vi "Client Download and Print PDF.vi"(8 "error in (no error)":errorcluster, 11 "PDF URL (\"\")":string) -> (0 "error out":errorcluster)   [LabVIEW 2011]
uses:
  Summitek EXT/Win32/WinSHELL/SHFolderPaths.ctl
  Spartan Client Version.vi
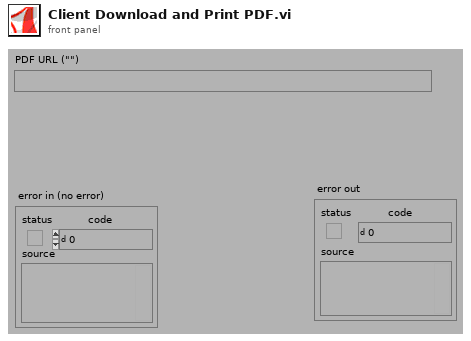
[diagram p1: front panel]
types:
  T1 = typedef "SHFolderPaths.ctl" = i32
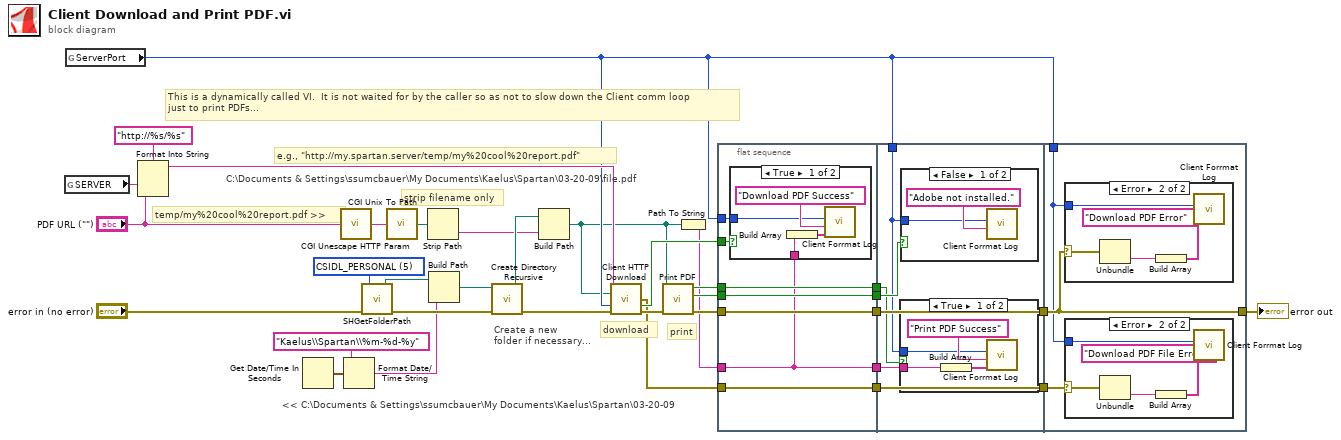
[diagram p0: block diagram]
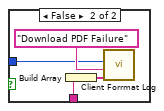
[diagram p2: hidden frame]
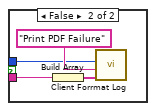
[diagram p3: hidden frame]
diagram:
  w34 = T1 5 items=["CSIDL_DESKTOP"=0, "CSIDL_PERSONAL"=5, "CSIDL_STARTUP"=7, "CSIDL_BITBUCKET"=10, "CSIDL_DRIVES"=17, "CSIDL_NETWORK"=18, "CSIDL_COMMON_PROGRAMS"=23, "CSIDL_COMMON_STARTUP"=24, "CSIDL_COMMON_DESKTOPDIRECTORY"=25, "CSIDL_PROGRAM_FILES"=38] ("Shell Folder (DESKTOP)")
  # "print"
  # "temp/my%20cool%20report.pdf >>"
  # "strip filename only"
  # "e.g., \"http://my.spartan.server/temp/my%20cool%20report.pdf\""
  # "download"
  # "This is a dynamically called VI.  It is not waited for by the caller so as not to slow down the Client comm loop\njust to print PDFs..."
  # "<< C:\\Documents & Settings\\ssumcbauer\\My Documents\\Kaelus\\Spartan\\03-20-09"
  # "C:\\Documents & Settings\\ssumcbauer\\My Documents\\Kaelus\\Spartan\\03-20-09\\file.pdf"
  # "Create a new\nfolder if necessary..."
  n1 = global read "Spartan Client Version.vi" "SERVER"() -> (w7:string)
  n2 = global read "Spartan Client Version.vi" "ServerPort"() -> (w6:u16)
  n3 = Format Into String(format string="http://%s/%s" ("name (unnamed)"), w7, "PDF URL (\"\")") -> (resulting string=w22:string)  [unwired: 2 in, 1 out]
  n4 = Get Date/Time In Seconds() -> (seconds since 1Jan1904=w31:timestamp)
  n5 = call "CGI Unescape HTTP Param.vi"("url-encoded string"="PDF URL (\"\")") -> ("string"=w19:string)
  n6 = Format Date/Time String(time format string (%c)="Kaelus\\Spartan\\%m-%d-%y", seconds (now)=w31) -> (date/time string=w29:string)  [unwired: 1 out]
  n7 = call "SHGetFolderPath.vi"("error in (no error)"="error in (no error)", "Shell Folder (DESKTOP)"=w34) -> ("error out"=w33:errorcluster, "FolderPath"=w32:path)  [unwired: 4 out]
  n8 = call "CGI Unix To Path.vi"("unix path"=w19) -> ("platform path"=w24:path)  [unwired: 1 out]
  n9 = Strip Path(path=w24) -> (name=w21:string)  [unwired: 1 out]
  n10 = Build Path(base path=w32, name or relative path=w29) -> (appended path=w28:path)
  n11 = call <vilib>:"Create Directory Recursive.vi"("error in (no error)"=w33, "directory"=w28) -> ("error out"=w26:errorcluster, "directory copy"=w27:path)  [unwired: 1 in, 3 out]
  n12 = Build Path(base path=w27, name or relative path=w21) -> (appended path=w5:path)
  n13 = call "Client HTTP Download.vi"("http URL"=w22, "file path (Not A Path)"=w5, "Port (80)"=w6, "error in (no error)"=w26) -> ("file error"=w12:errorcluster, "success"=w18:bool, "error out"=w25:errorcluster)  [unwired: 1 in, 8 out]
  n14 = call "Print PDF.vi"("error in (no error)"=w25, "PDF Path"=w5) -> ("error out"=w16:errorcluster, "Adobe Installed?"=w13:bool, "Printed?"=w3:bool)  [unwired: 7 out]
  n15 = Path To String(path=w5) -> (string=w1:string)
  n16 = flat-sequence {
    tunnel: w18 -> [w41]
    tunnel: [w40] -> w17
    tunnel: w16 -> [w40]
    tunnel: [w39] -> w14
    tunnel: w13 -> [w39]
    tunnel: w12 -> [w38]
    tunnel: [w38] -> w11
    tunnel: w6 -> [w37]
    tunnel: [w36] -> w4
    tunnel: w3 -> [w36]
    tunnel: [w35] -> w2
    tunnel: w1 -> [w35]
    tunnel: w17 -> [w55]
    tunnel: [w55] -> w15
    tunnel: w14 -> [w54]
    tunnel: w11 -> [w53]
    tunnel: [w53] -> w10
    tunnel: w6 -> [w51]
    tunnel: w4 -> [w52]
    tunnel: w2 -> [w50]
    tunnel: w15 -> [w68]
    tunnel: [w68] -> w9
    tunnel: w10 -> [w67]
    tunnel: w6 -> [w66]
    frame #0 {
      n17 = case shown="True" w41 {
        tunnel: w37 -> [w43 w48]
        tunnel: w35 -> [w42 w46]
        frame True {
          n18 = Build Array(w42) -> (w44:string[])
          n19 = call "Client Forrmat Log.vi"("Params (empty)"=w44, "Command (\"\")"="Download PDF Success", "ServerPort (80)"=w43) -> ()  [unwired: 1 in, 8 out]
        }
        frame False {
          n20 = Build Array(w46) -> (w47:string[])
          n21 = call "Client Forrmat Log.vi"("Params (empty)"=w47, "Command (\"\")"="Download PDF Failure", "ServerPort (80)"=w48) -> ()  [unwired: 1 in, 8 out]
        }
      }
    }
    frame #1 {
      n22 = case shown="True" w52 {
        tunnel: w51 -> [w57 w61]
        tunnel: w50 -> [w56 w60]
        frame True {
          n23 = Build Array(w56) -> (w58:string[])
          n24 = call "Client Forrmat Log.vi"("Params (empty)"=w58, "Command (\"\")"="Print PDF Success", "ServerPort (80)"=w57) -> ()  [unwired: 1 in, 8 out]
        }
        frame False {
          n25 = Build Array(w60) -> (w62:string[])
          n26 = call "Client Forrmat Log.vi"("Params (empty)"=w62, "Command (\"\")"="Print PDF Failure", "ServerPort (80)"=w61) -> ()  [unwired: 1 in, 8 out]
        }
      }
      n27 = case shown="False" w54 {
        tunnel: w51 -> [w64 _]
        frame False {
          n28 = call "Client Forrmat Log.vi"("Command (\"\")"="Adobe not installed.", "ServerPort (80)"=w64) -> ()  [unwired: 2 in, 8 out]
        }
        frame True {
        }
      }
    }
    frame #2 {
      n29 = case shown="Error" w68 {
        selector: w68 -> [_ w78]
        tunnel: w66 -> [_ w74]
        frame No Error {
        }
        frame Error {
          n30 = Unbundle(w78) -> ("source"=w77:string)  [unwired: 2 out]
          n31 = Build Array(w77) -> (w75:string[])
          n32 = call "Client Forrmat Log.vi"("Params (empty)"=w75, "Command (\"\")"="Download PDF Error", "ServerPort (80)"=w74) -> ()  [unwired: 1 in, 8 out]
        }
      }
      n33 = case shown="Error" w67 {
        selector: w67 -> [_ w73]
        tunnel: w66 -> [_ w69]
        frame No Error {
        }
        frame Error {
          n34 = Unbundle(w73) -> ("source"=w72:string)  [unwired: 2 out]
          n35 = Build Array(w72) -> (w70:string[])
          n36 = call "Client Forrmat Log.vi"("Params (empty)"=w70, "Command (\"\")"="Download PDF File Error", "ServerPort (80)"=w69) -> ()  [unwired: 1 in, 8 out]
        }
      }
    }
  }
  "error out" <- w9
